vi "GetAllAnalogInputVals.vi"(8 "error in (no error)":errorcluster, 11 "SerialPortRef":T1) -> (0 "error out":errorcluster, 1 "ADC raw values":u32[](array[numeric]) format="%012b", 2 "ADC voltages":dbl[](array[numeric]), 3 "SerialPortRef 2":T1)   [LabVIEW 2015]
uses:
  <vilib>/Rock Robotics/WPI/SerialPort/WPI_SerialPortRef.ctl
panel:
  out "Full String Recieved":string
  out "Recieved Checksum":string
  out "Calculated Checksum":string
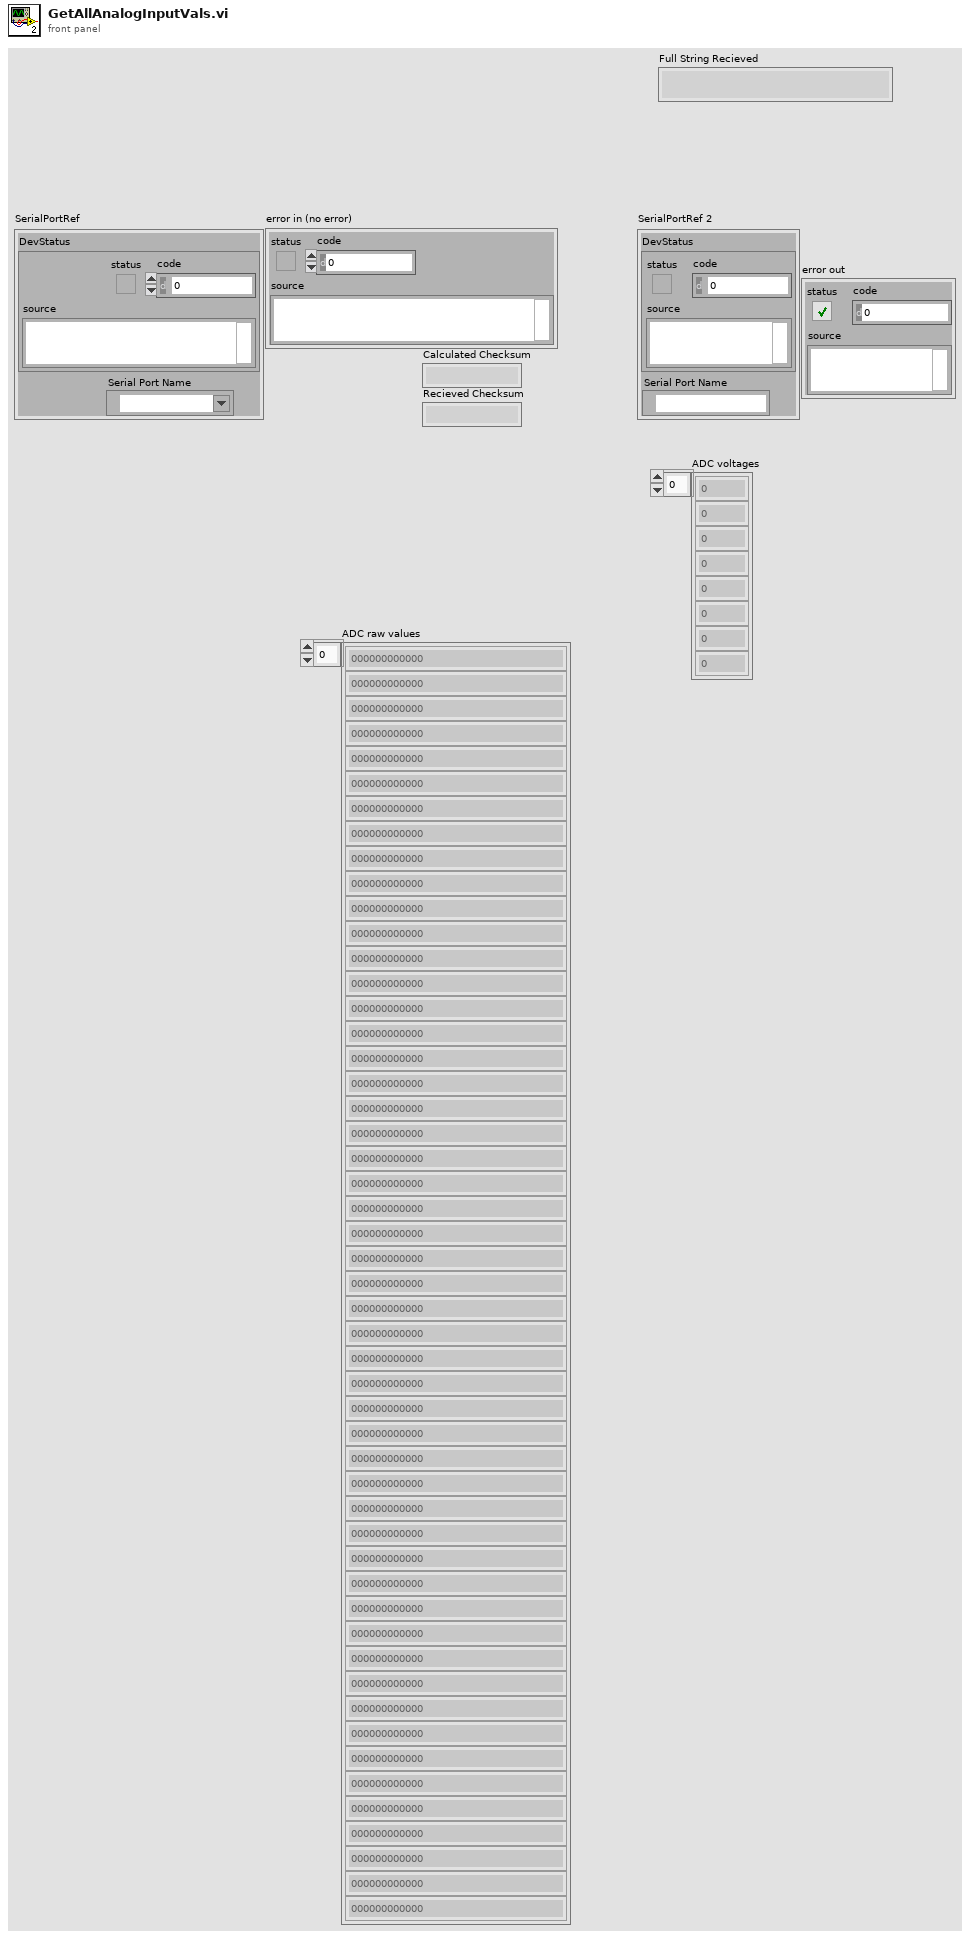
[diagram p1: front panel]
types:
  T1 = typedef "WPI_SerialPortRef.ctl" = cluster{"DevStatus":errorcluster, "Serial Port Name":refnum<visa-resource-name>}
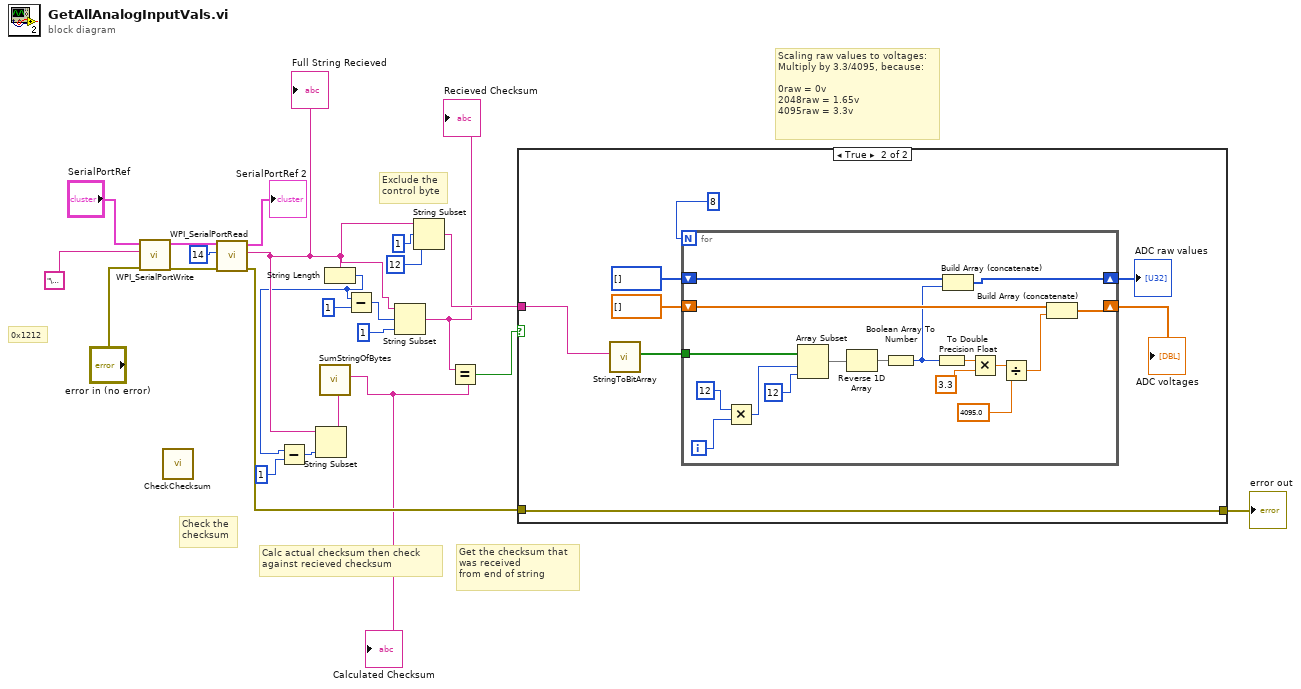
[diagram p0: block diagram]
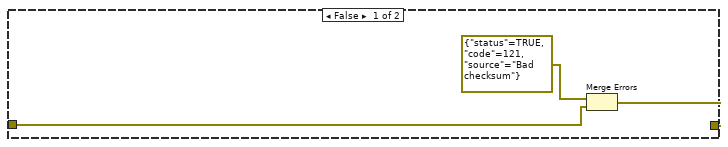
[diagram p2: hidden frame]
diagram:
  # "Exclude the \ncontrol byte"
  # "Calc actual checksum then check \nagainst recieved checksum"
  # "Get the checksum that\nwas received \nfrom end of string"
  # "Scaling raw values to voltages:\nMultiply by 3.3/4095, because:\n\n0raw = 0v\n2048raw = 1.65v\n4095raw = 3.3v"
  # "Check the\nchecksum"
  # "0x1212"
  n1 = call <vilib>:"WPI_SerialPortWrite.vi"("error in (no error)"="error in (no error)", "Buffer"="\u0012", "SerialPortRef"="SerialPortRef") -> ("error out"=w14:errorcluster, "SerialPortRef"=w15:T1)  [unwired: 6 in, 1 out]
  n2 = call "CheckChecksum.vi"() -> ()  [unwired: 10 in, 2 out]
  n3 = call <vilib>:"WPI_SerialPortRead.vi"("error in (no error)"=w14, "Num Bytes to Read"=u32 14, "SerialPortRef"=w15) -> ("error out"=w12:errorcluster, "Buffer"=w4:string, "SerialPortRef"=→"SerialPortRef 2":T1)  [unwired: 6 in]
  "Full String Recieved" <- w4
  n4 = String Length(string=w4) -> (length=w3:i32)
  n5 = Subtract(x=w3, y=1) -> (x-y=w2:i32)
  n6 = String Subset(string=w4, length (rest)=w2) -> (substring=w5:string)  [unwired: 1 in]
  n7 = call "SumStringOfBytes.vi"("String Of Bytes"=w5) -> ("SumAsString"=w8:string)  [unwired: 10 in]
  "Calculated Checksum" <- w8
  n8 = Subtract(x=w3, y=1) -> (x-y=w10:i32)
  n9 = String Subset(string=w4, offset (0)=w10, length (rest)=1 ("length (rest)")) -> (substring=w6:string)
  "Recieved Checksum" <- w6
  n10 = String Subset(string=w4, offset (0)=1, length (rest)=12 ("length (rest)")) -> (substring=w19:string)
  n11 = Equal?(x=w6, y=w8) -> (x = y?=w7:bool)
  n12 = case shown="True" w7 {
    tunnel: w19 -> [_ w29]
    tunnel: w12 -> [w25 w34]
    tunnel: [w24 w34] -> w18
    frame False {
      n13 = Merge Errors(errorcluster {"status"=TRUE, "code"=121, "source"="Bad checksum"} ("error in"), w25) -> (w24:errorcluster)
    }
    frame True {
      n14 = call "StringToBitArray.vi"("string"=w29) -> ("Array"=w32:bool[])  [unwired: 10 in]
      n15 = for {
        N: 8 -> [_]
        tunnel: w32 -> [w51]
        shift-right: [w47] -> w30
        shift-left: u32[] [] -> [w46]
        shift-right: [w42] -> w27
        shift-left: dbl[] [] -> [w41]
        i -> [w50]
        n16 = Multiply(x=12, y=w50) -> (x*y=w48:i32)
        n17 = Array Subset(array=w51, index=w48, length=12) -> (w44:bool[])
        n18 = Reverse 1D Array(array=w44) -> (reversed array=w43:bool[])
        n19 = Boolean Array To Number(Boolean array=w43) -> (number=w35:u32)
        n20 = To Double Precision Float(number=w35) -> (double precision float=w36:dbl)
        n21 = Build Array (concatenate)(w46, w35) -> (w47:u32[])
        n22 = Multiply(x=w36, y=3.3) -> (x*y=w39:dbl)
        n23 = Divide(x=w39, y=4095.0) -> (x/y=w37:dbl)
        n24 = Build Array (concatenate)(w41, w37) -> (w42:dbl[])
      }
      "ADC raw values" <- w30
      "ADC voltages" <- w27
    }
  }
  "error out" <- w18
